vi "20211008_HW02.vi"() -> ()   [LabVIEW 2019]
panel:
  out "Number of True":i32
  in  "Array":i32[](array[numeric])
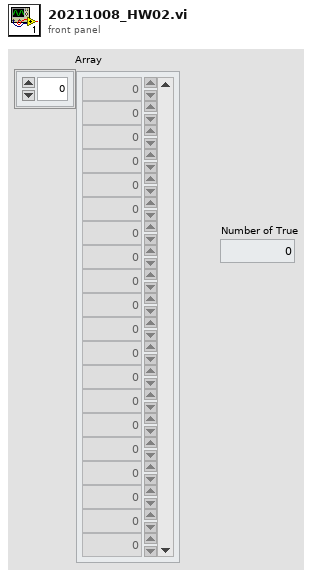
[diagram p1: front panel]
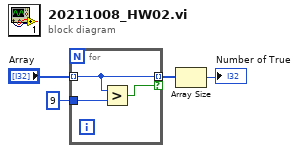
[diagram p0: block diagram]
diagram:
  n1 = for {
    tunnel: "Array" -> [w7] mode=indexing
    tunnel: [w7] -> w3 mode=indexing if=w6
    tunnel: 9 ("y") -> [w5]
    n2 = Greater?(x=w7, y=w5) -> (0:w6:bool)
  }
  n3 = Array Size(array=w3) -> (size(s)=→"Number of True":i32)
